vi "Launch Nested Process.vi"(8 "error in (no error)":errorcluster, 10 "Nested":refnum<class "CoolAppProcess.lvclass">, 11 "CoolAppProcess in":refnum<class "CoolAppProcess.lvclass">) -> (0 "error out":errorcluster, 2 "Enqr":refnum<class "Message Enqueuer.lvclass">, 3 "CoolAppProcess out":refnum<class "CoolAppProcess.lvclass">)   [LabVIEW 2020, in "LAF2024Q2.lvlib" / "CoolAppProcess.lvclass"]
uses:
  CoolAppProcess.lvclass
  C:/Program Files (x86)/National Instruments/LabVIEW 2020/vi.lib/ActorFramework/Actor/Actor.lvclass
  <vilib>/ActorFramework/Message Enqueuer/Message Enqueuer.lvclass
  CoolAppProcess.lvclass/CoolAppProcess.ctl
  <vilib>/ActorFramework/Actor/Actor.lvclass
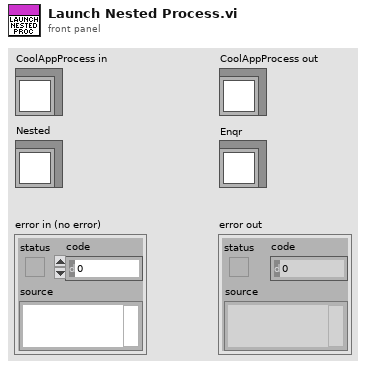
[diagram p1: front panel]
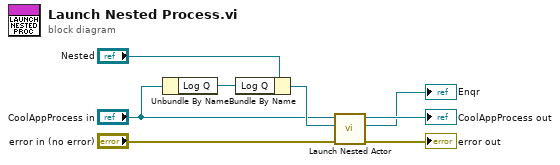
[diagram p0: block diagram]
diagram:
  n1 = Unbundle By Name("CoolAppProcess in") -> ("Log Q"=w2:refnum<queue>)
  n2 = Bundle By Name(cluster="Nested", "Log Q"=w2) -> (w4:refnum<class "CoolAppProcess.lvclass">)
  n3 = call <vilib>:"Launch Nested Actor.vi"("error in (no error)"="error in (no error)", "Nested Actor"=w4, "Caller Actor in"="CoolAppProcess in") -> ("error out"=→"error out":errorcluster, "Nested Actor's Enqueuer"=→"Enqr":refnum<class "Message Enqueuer.lvclass">, "Caller Actor out"=→"CoolAppProcess out":refnum<class "CoolAppProcess.lvclass">)  [unwired: 6 in]
